vi "Configure Maximum Length Sequence.vi"(0 "template configuration":refnum<class "SV Signal.lvclass">, 5 "polynomial order":i32=31, 7 "amplitude":dbl=1.0, 9 "seed":i64=-1, 11 "error in (no error)":errorcluster) -> (4 "signal configuration":refnum<class "SV MLS.lvclass">, 15 "error out":errorcluster)   [LabVIEW 2017, in "SV MLS.lvclass"]
doc: "Configures a user-defined test signal. Wire the outputs to SV Signal (waveform) VI to generate the test signal, or wire to SV Signal Property Node to configure additional parameters before wiring to the SV Signal (waveform) VI."
uses:
  <vilib>/addons/_NISVFA/_Generation/Signal Generation/SV MLS/SV MLS.lvclass
  C:/Program Files (x86)/National Instruments/LabVIEW 2017/vi.lib/addons/_NISVFA/_Generation/Signal Generation/SV Signal/SV Signal.lvclass
  <vilib>/addons/_NISVFA/_Generation/Signal Generation/SV Signal/SV Signal.lvclass
  <vilib>/addons/_NISVFA/_Generation/Signal Generation/SV MLS/SV MLS.lvclass/SV MLS.ctl
  <vilib>/addons/_NISVFA/_Generation/Signal Generation/SV Signal/Write Post-Measurement Settling Duration.vi
  <vilib>/addons/_NISVFA/_Generation/Signal Generation/SV Signal/Write Pre-Measurement Settling Duration.vi
  <vilib>/addons/_NISVFA/_Generation/Signal Generation/SV Signal/Write Measurement Duration.vi
  <vilib>/addons/_NISVFA/_Generation/Signal Generation/SV Signal/Write Sample Rate.vi
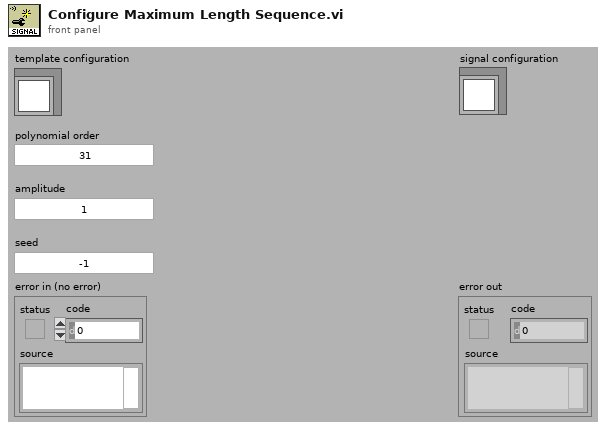
[diagram p1: front panel]
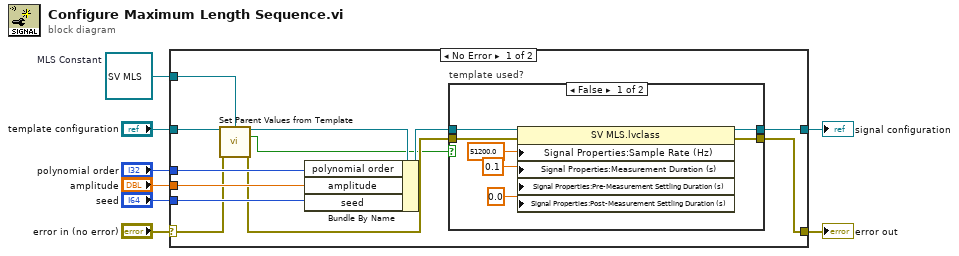
[diagram p0: block diagram]
diagram:
  w6 = refnum<class "SV MLS.lvclass"> refnum  # MLS Constant
  n1 = case shown="No Error" "error in (no error)" {
    selector: "error in (no error)" -> [w11 w30]
    tunnel: [w16 w30] -> w7
    tunnel: [w15 w31] -> w3
    tunnel: w6 -> [w13 w31]
    tunnel: "amplitude" -> [w20 _]
    tunnel: "seed" -> [w19 _]
    tunnel: "polynomial order" -> [w18 _]
    tunnel: "template configuration" -> [w14 _]
    frame No Error {
      n2 = call-dynamic "Set Parent Values from Template.vi"("template configuration"=w14, "signal configuration in"=w13, "error in (no error)"=w11) -> ("signal configuration out"=w12:refnum<class "SV MLS.lvclass">, "template used?"=w9:bool, "error out"=w10:errorcluster)  [unwired: 10 in]
      n3 = Bundle By Name(cluster=w12, "polynomial order"=w18, "amplitude"=w20, "seed"=w19) -> (w17:refnum<class "SV MLS.lvclass">)
      n4 = case "template used?" shown="False" w9 {
        tunnel: w17 -> [w24 w29]
        tunnel: [w23 w28] -> w16
        tunnel: [w22 w29] -> w15
        tunnel: w10 -> [w21 w28]
        frame False {
          w27 = 0.0 ("settling time_s")
          n5 = property class="SV MLS.lvclass"(reference=w24, error in=w21, "Signal Properties:Sample Rate (Hz)"=51200.0 ("SampleRate_Hz"), "Signal Properties:Measurement Duration (s)"=0.1 ("integration time_s"), "Signal Properties:Pre-Measurement Settling Duration (s)"=w27, "Signal Properties:Post-Measurement Settling Duration (s)"=w27) -> (reference out=w22:refnum<class "SV MLS.lvclass">, error out=w23:errorcluster)
        }
        frame True {
        }
      }
    }
    frame Error {
    }
  }
  "error out" <- w7
  "signal configuration" <- w3
